vi "SwissSPAD Live_Special Controls Update.vi"(7 "Verbose (T)":bool=TRUE, 8 "error in (no error)":errorcluster, 9 "Settings List Element":T1, 11 "VI Refnum":refnum<vi>) -> (0 "Error Out":errorcluster)   [LabVIEW 2021]
uses:
  SwissSPAD Live_Settings List.ctl
  SwissSPAD Live_Settings Q Element.ctl
  SwissSPAD Live_Settings Q Action.ctl
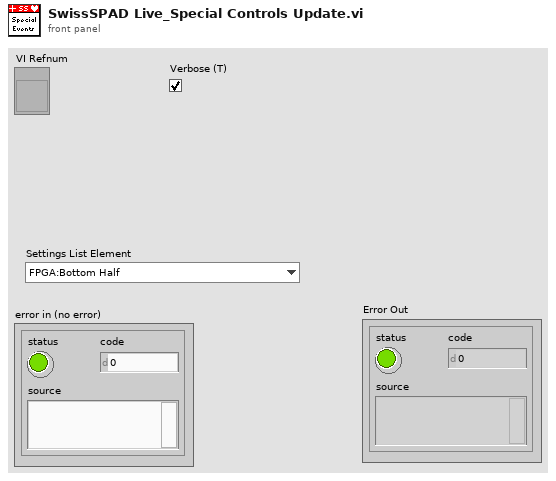
[diagram p1: front panel]
types:
  T1 = typedef "SwissSPAD Live_Settings List.ctl" = enum16{"FPGA:Bottom Half", "FPGA:Top Half", "FPGA:Bottom Bitfile Path", "FPGA:Top Bitfile Path", "FPGA:Bottom Bitstream Version", "FPGA:Top Bitstream Version", "FPGA:Auto Reset FPGA", "FPGA:Bottom FPGA Serial Number", "FPGA:Top FPGA Serial Number", "FPGA:Detector PCB Version", "Acquisition Parameters:Microlens", "Acquisition Parameters:SS2 DAQ Parameters", "Acquisition Parameters:Gate Configuration Array", "Acquisition Parameters:SS3 DAQ Parameters", "Acquisition Parameters:Buffer Size (# 8-bit Gates)", "File Information:File Information", "File Information:# Datasets in Series", "File Information:Scrambled File Flag", "File Information:SS3 Gate Slip Correction", "File Information:SS3 Hot Pixel Mismatch Detection", "File Information:Delay between Datasets", "File Information:Save Sum of All Gates Preview", "Image Parameters:Image ROI Information", "Image Parameters:Image Binning Options", "Image Parameters:SS3 Displayed Image", "Image Parameters:Image Display Options", "Image Parameters:Use Histogram Cursors", "Image Parameter:FPGA Data to Display", "UI Settings:Histogram Bins Number", "UI Settings:Histogram Bin Size", "UI Settings:Use Image Display Options", "UI Settings:Verbose Settings", "UI Settings:Verbose Saving"}
  T2 = typedef "SwissSPAD Live_Settings Q Element.ctl" = cluster{"Action":T3, "Data":variant}
  T3 = typedef "SwissSPAD Live_Settings Q Action.ctl" = enum16{"Idle", "Initialization", "Refresh All Parameters", "Store Current Configuration", "Rename Current Configuration", "Delete Current Configuration", "Update Image ROI Information", "Load Hot Pixel Mask Image", "Quit"}
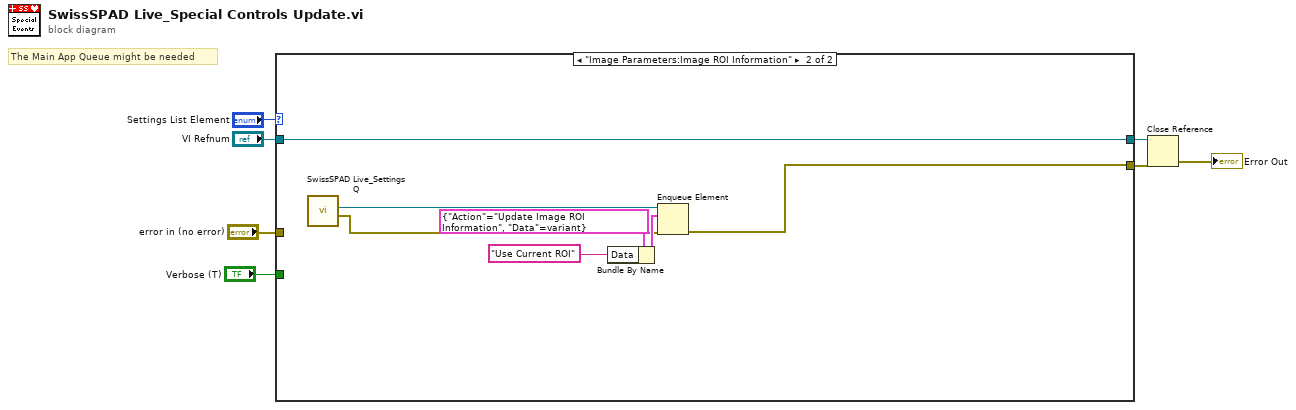
[diagram p0: block diagram]
diagram:
  # "The Main App Queue might be needed"
  n1 = case shown="\"Image Parameters:Image ROI Information\"" "Settings List Element" {
    tunnel: "VI Refnum" -> [w9 w16]
    tunnel: "error in (no error)" -> [w8 _]
    tunnel: [w9 w16] -> w4
    tunnel: [w8 w12] -> w2
    tunnel: "Verbose (T)" -> [_ _]
    frame "FPGA:Bottom Half", Default {
    }
    frame "Image Parameters:Image ROI Information" {
      n2 = call "SwissSPAD Live_Settings Q.vi"() -> ("error out"=w10:errorcluster, "Queue out"=w11:refnum<queue>)  [unwired: 10 in]
      n3 = Bundle By Name(cluster=T2 {"Action"=enum."Update Image ROI Information", "Data"=variant} ("element"), "Data"="Use Current ROI") -> (w14:T2)
      n4 = Enqueue Element(queue=w11, element=w14, error in (no error)=w10) -> (error out=w12:errorcluster)  [unwired: 1 in, 2 out]
    }
  }
  n5 = Close Reference(reference=w4, error in (no error)=w2) -> (error out=→"Error Out":errorcluster)
